vi "p2.vi"() -> ()   [LabVIEW 2023, in "d5.lvlib"]
uses:
  d5.lvlib
  <vilib>/regexp/Match Regular Expression.xnode
  AOC/AOC.lvlib
panel:
  out "Answer":i64
  in  "Example":string="seeds: 79 14 55 13\n\nseed-to-soil map:\n50 98 2\n52 50 48\n\nsoil-to-fertilizer map:\n0 15 37\n37 52 2\n39 0 15\n\nfertilizer-to-water map:\n49 53 8\n0 11 42\n42 0 7\n57 7 4\n\nwater-to-light map:\n88 18 7\n18 25 70\n\nlight-to-temperature map:\n45 77 23\n81 45 19\n68 64 13\n\ntemperature-to-humidity map:\n0 69 1\n1 0 69\n\nhumidity-to-location map:\n60 56 37\n56 93 4"
  in  "Example":bool
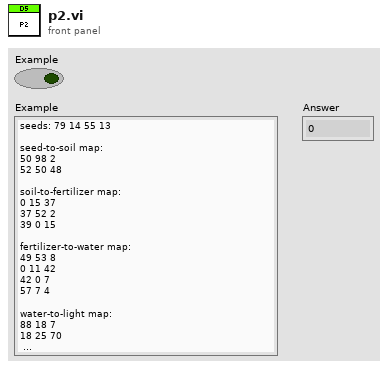
[diagram p1: front panel]
types:
  T1 = cluster{cluster{"dst":i64, "src":i64, "rng":i64}[]}
  T2 = cluster{cluster{"dst":i64, "src":i64, "rng":i64}[]}[]
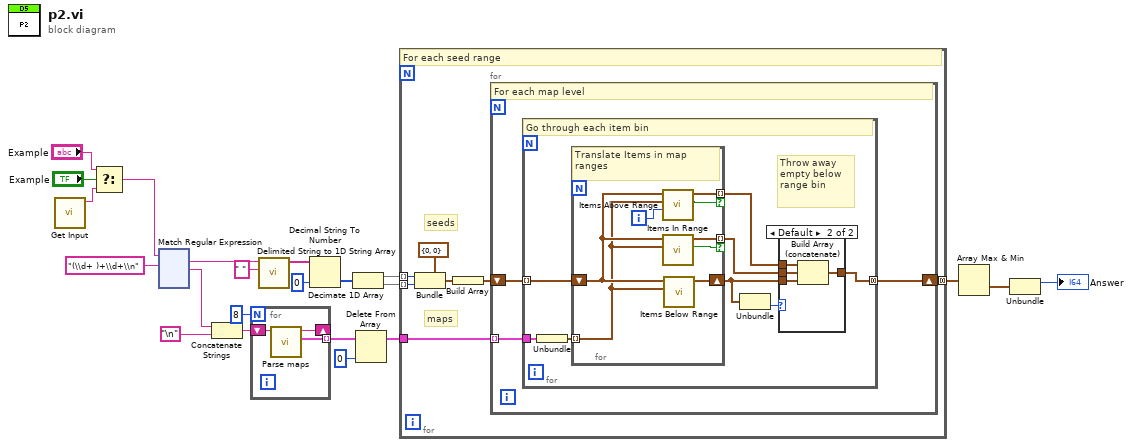
[diagram p0: block diagram]
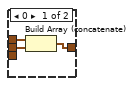
[diagram p2: hidden frame]
diagram:
  n1 = call "Get Input.vi"() -> ("Input"=w22:string)  [unwired: 11 in]
  n2 = Select(t="Example", s="Example", f=w22) -> (s? t:f=w14:string)
  n3 = xnode "Match Regular Expression"("input string"=w14, "regular expression"="(\\d+ )+\\d+\\n") -> ("whole match"=w13:string, "after match"=w12:string)  [unwired: 4 in, 3 out]
  n4 = Concatenate Strings(w12, "\n") -> (w16:string)
  n5 = for {
    N: 8 -> [_]
    shift-right: [w24] -> _
    shift-left: w16 -> [w25]
    tunnel: [w23] -> w10 mode=indexing
    n6 = call "Parse maps.vi"("string in"=w25) -> ("map"=w23:T1, "string out"=w24:string)  [unwired: 9 in]
  }
  n7 = call <vilib>:"Delimited String to 1D String Array.vi"("delimiter"=" ", "delimited string"=w13) -> ("string array"=w11:string[])  [unwired: 9 in]
  n8 = Decimal String To Number(string=w11, default (0L)=i64 0 ("default (0 I32)")) -> (number=w5:i64[])  [unwired: 1 in, 1 out]
  n9 = Decimate 1D Array(w5) -> (w4:i64[], w3:i64[])
  n10 = Delete From Array(array=w10, index=0) -> (array with subset deleted=w9:T2)  [unwired: 1 in, 1 out]
  n11 = for {
    tunnel: w9 -> [w32]
    tunnel: [w31] -> w7 mode=concatenating
    tunnel: w4 -> [w28] mode=indexing
    tunnel: w3 -> [w27] mode=indexing
    # "seeds"
    # "maps"
    # "For each seed range"
    n12 = Bundle(cluster=cluster{"strt":i64, "rng":i64} {"strt"=0, "rng"=0}, "strt"=w28, "rng"=w27) -> (w26:cluster{"strt":i64, "rng":i64})
    n13 = Build Array(w26) -> (w30:cluster{"strt":i64, "rng":i64}[])
    n14 = for {
      tunnel: w32 -> [w35] mode=indexing
      shift-right: [w33] -> w31
      shift-left: w30 -> [w34]
      # "For each map level"
      n15 = for {
        tunnel: w35 -> [w43]
        tunnel: w34 -> [w40] mode=indexing
        tunnel: [w41] -> w33 mode=concatenating
        # "Throw away empty below range bin"
        # "Go through each item bin"
        n16 = Unbundle(w43) -> (w42:cluster{"dst":i64, "src":i64, "rng":i64}[])
        n17 = for {
          tunnel: w42 -> [w45] mode=indexing
          tunnel: [w48] -> w39 mode=indexing if=w44
          tunnel: [w50] -> w38 mode=indexing if=w51
          shift-right: [w49] -> w37
          shift-left: w40 -> [w46]
          i -> [w47]
          # "Translate Items in map ranges"
          n18 = call "Items Above Range.vi"("map index"=w47, "Location Translation"=w45, "Initial Items"=w46) -> ("Keep Items?"=w44:bool, "Items Above Range"=w48:cluster{i64, "lower limit":i64})  [unwired: 7 in]
          n19 = call "Items In Range.vi"("Location Translation"=w45, "Initial Items"=w46) -> ("Keep?"=w51:bool, "Items In Range"=w50:cluster{i64, "upper limit":i64})  [unwired: 8 in]
          n20 = call "Items Below Range.vi"("Location Translation"=w45, "Initial Items"=w46) -> ("Items Below Range"=w49:cluster{"strt":i64, "rng":i64})  [unwired: 9 in]
        }
        n21 = Unbundle(w37) -> ("rng"=w36:i64)  [unwired: 1 out]
        n22 = case shown="Default" w36 {
          tunnel: [w52 w58] -> w41
          tunnel: w39 -> [w54 w57]
          tunnel: w38 -> [w53 w56]
          tunnel: w37 -> [_ w55]
          frame 0 {
            n23 = Build Array (concatenate)(w54, w53) -> (w52:cluster{i64, "upper limit":i64}[])
          }
          frame Default {
            n24 = Build Array (concatenate)(w57, w56, w55) -> (w58:cluster{"strt":i64, "rng":i64}[])
          }
        }
      }
    }
  }
  n25 = Array Max & Min(array=w7) -> (min value=w2:cluster{"strt":i64, "rng":i64})  [unwired: 3 out]
  n26 = Unbundle(w2) -> ("strt"=→"Answer":i64)  [unwired: 1 out]
